vi "MSGR Elements in Q.vi"(1 "MSGR Q name":T1, 11 "error in (no error)":errorcluster) -> (6 "# elements in queue":i32, 15 "error out":errorcluster)   [LabVIEW 2018]
doc: "$Author::Richard Jennings $\n$Rev:: $\n$Date:: May, 2008 $\n\nOVERVIEW:\nReentrant VI to receive messages via a MSGR Q. If the Q does not exist this VI will create it, then wait for data.\n\nINPUTS (Controls):\n<name> - <short description of each control wired to connector pane>\n\nOUTPUTS (Indicators):\n<name> - <short description of each indicator wired to connector pane>\n\nCopyright 2008 - 2017 Jennings Embedded Servies. All rights reserved.\nAuthor makes no warranties or guarantees related to performance of the software.\nUSE AT YOUR OWN RISK\nwww.jembedded.com\n\n\n\nMIT License\n\nCopyright (c) 2020 RichardLGP5\n\nPermission is hereby granted, free of charge, to any person obtaining a copy\nof this software and associated documentation files (the \"Software\"), to deal\nin the Software without restriction, including without limitation the rights\nto use, copy, modify, merge, publish, distribute, sublicense, and/or sell\ncopies of the Software, and to permit persons to whom the Software is\nfurnished to do so, subject to the following conditions:\n\nThe above copyright notice and this permission notice shall be included in all\ncopies or substantial portions of the Software.\n\nTHE SOFTWARE IS PROVIDED \"AS IS\", WITHOUT WARRANTY OF ANY KIND, EXPRESS OR\nIMPLIED, INCLUDING BUT NOT LIMITED TO THE WARRANTIES OF MERCHANTABILITY,\nFITNESS FOR A PARTICULAR PURPOSE AND NONINFRINGEMENT. IN NO EVENT SHALL THE\nAUTHORS OR COPYRIGHT HOLDERS BE LIABLE FOR ANY CLAIM, DAMAGES OR OTHER\nLIABILITY, WHETHER IN AN ACTION OF CONTRACT, TORT OR OTHERWISE, ARISING FROM,\nOUT OF OR IN CONNECTION WITH THE SOFTWARE OR THE USE OR OTHER DEALINGS IN THE\nSOFTWARE."
uses:
  MSGR Q Name TypeDef.ctl
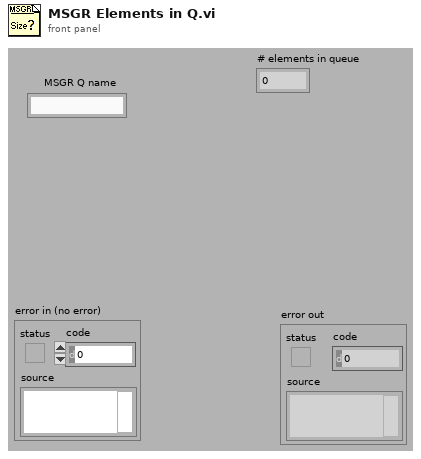
[diagram p1: front panel]
types:
  T1 = typedef "MSGR Q Name TypeDef.ctl" = string
  T2 = typedef "MSGR Q Ref TypeDef.ctl" = refnum<queue>
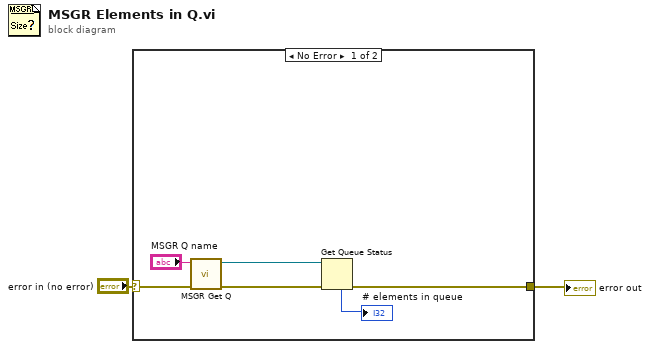
[diagram p0: block diagram]
diagram:
  n1 = case shown="No Error" "error in (no error)" {
    selector: "error in (no error)" -> [w8 w9]
    tunnel: [w5 w9] -> w2
    frame No Error {
      n2 = call "MSGR Get Q.vi"("error in (no error)"=w8, "MSGR Q name"="MSGR Q name") -> ("error out"=w4:errorcluster, "MSGR Q"=w6:T2)  [unwired: 8 out]
      n3 = Get Queue Status(queue=w6, error in (no error)=w4) -> (error out=w5:errorcluster, # elements in queue=→"# elements in queue":i32)  [unwired: 1 in, 6 out]
    }
    frame Error {
    }
  }
  "error out" <- w2
